vi "Find All Systems.vi"(11 "Registered Systems":T3[](array[typedef])) -> (3 "Systems":T1[](array[typedef]))   [LabVIEW 2019]
uses:
  Type Defs and Controls/Registered System.ctl
  Type Defs and Controls/System Type.ctl
  Type Defs and Controls/System Cluster.ctl
  <vilib>/nisyscfg/Find Hardware.vi
  <vilib>/nisyscfg/Close (System).vi
  <resource>/objmgr/daqmx.rc
  <vilib>/nisyscfg/nisyscfg.lvlib
  <resource>/objmgr/nicontrollersysapi.rc
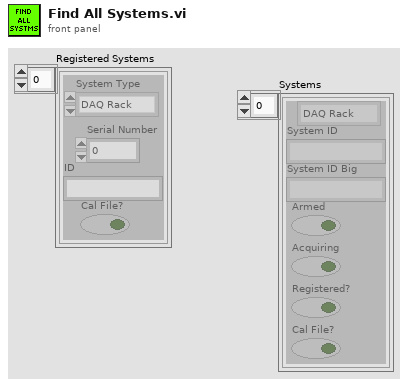
[diagram p1: front panel]
types:
  T1 = typedef "System Cluster.ctl" = cluster{"System Type":T2, "System ID":string, "System ID Big":string, "Armed":bool, "Acquiring":bool, "Registered?":bool, "Cal File?":bool}
  T2 = typedef "System Type.ctl" = enum16{"DAQ Rack", "DAQ Cart", "nx-5000", "unknown", "open"}
  T3 = typedef "Registered System.ctl" = cluster{"System Type":T2, "Serial Number":u32, "ID":string, "Cal File?":bool}
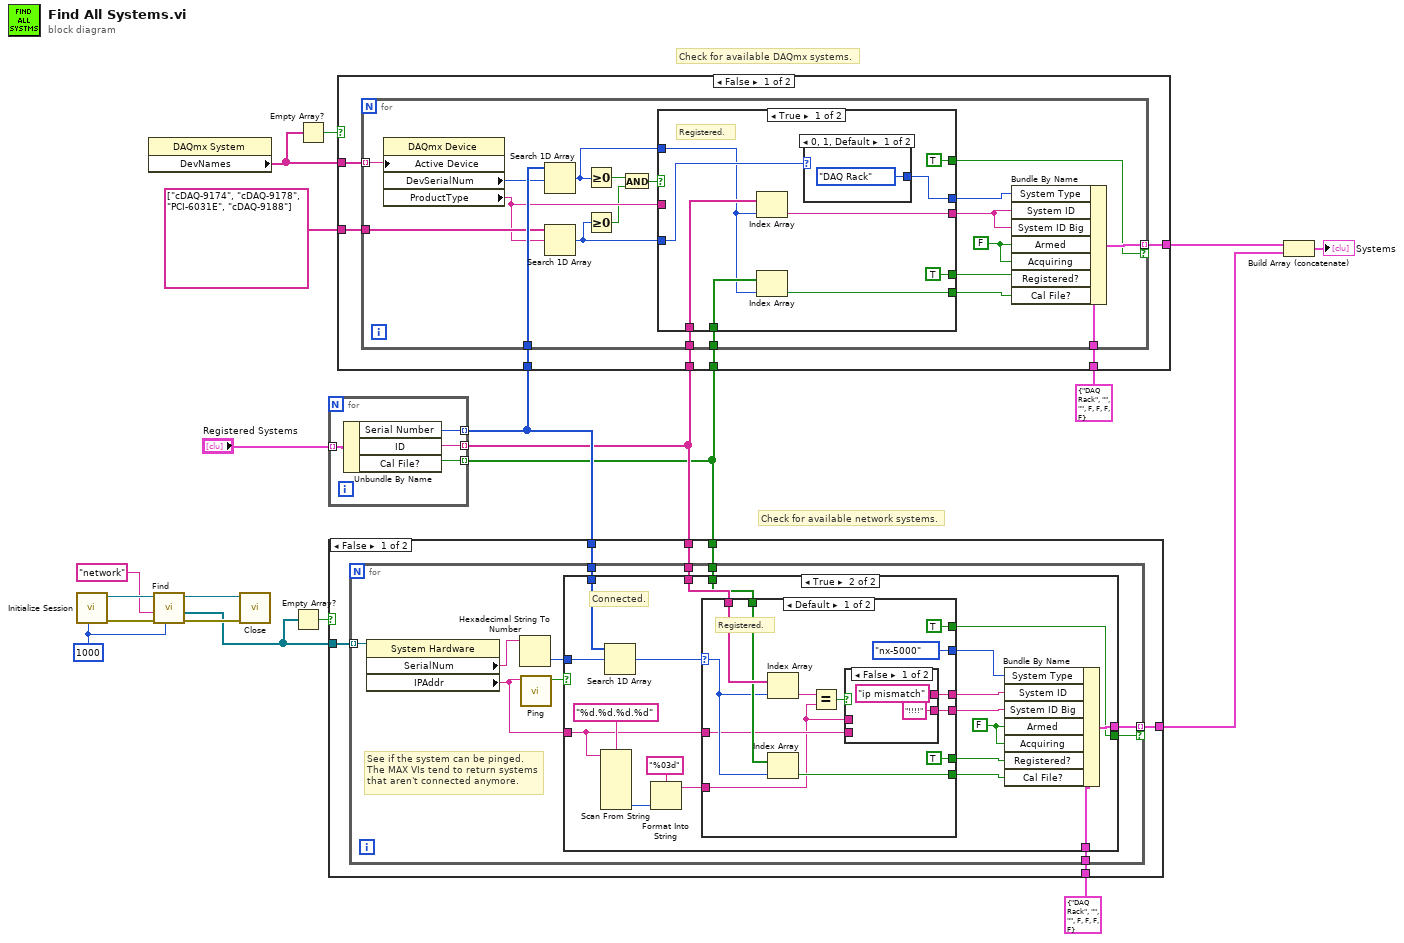
[diagram p0: block diagram]
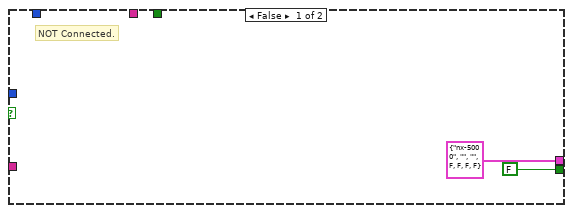
[diagram p2: hidden frame]
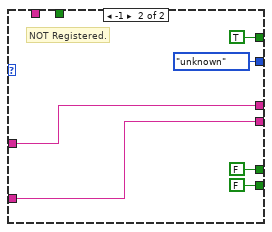
[diagram p4: hidden frame]
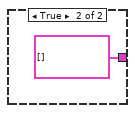
[diagram p5: hidden frame]
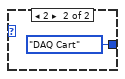
[diagram p6: hidden frame]
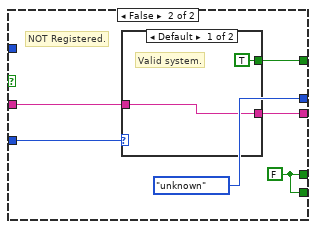
[diagram p7: hidden frame]
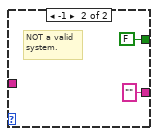
[diagram p8: hidden frame]
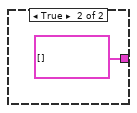
[diagram p9: hidden frame]
diagram:
  w15 = u32 1000 ("connect timeout in ms (4s)")
  # "Check for available network systems."
  # "Check for available DAQmx systems."
  n1 = call <vilib>:"Initialize Session.vi"("Connect Timeout (4000 ms)"=w15) -> ("error out"=w14:errorcluster, "Session out"=w11:refnum<k21>)  [unwired: 9 in]
  n2 = property class="DAQmx System"() -> ("DevNames"=w20:tag[])  [unwired: 2 in, 2 out]
  n3 = call-poly <vilib>:"Find.vi"("Remote Timeout (300,000 ms)"=w15, "error in (no error)"=w14, "Experts"="network" ("experts"), "Session in"=w11) -> ("error out"=w13:errorcluster, "Resources out"=w10:refnum<k20>[], "Session out"=w12:refnum<k21>)  [unwired: 4 in, 1 out]
  n4 = call-poly <vilib>:"Close.vi"("error in (no error)"=w13, "Session in"=w12) -> ()  [unwired: 9 in, 1 out]
  n5 = Empty Array?(array=w10) -> (empty?=w9:bool)
  n6 = Empty Array?(array=w20) -> (empty?=w19:bool)
  n7 = for {
    tunnel: "Registered Systems" -> [w24] mode=indexing
    tunnel: [w23] -> w8 mode=indexing
    tunnel: [w22] -> w6 mode=indexing
    tunnel: [w21] -> w5 mode=indexing
    n8 = Unbundle By Name(w24) -> ("Serial Number"=w23:u32, "ID"=w22:string, "Cal File?"=w21:bool)
  }
  n9 = case shown="False" w9 {
    tunnel: w10 -> [w30 _]
    tunnel: w8 -> [w29 _]
    tunnel: T1 {"System Type"=enum."DAQ Rack", "System ID"="", "System ID Big"="", "Armed"=FALSE, "Acquiring"=FALSE, "Registered?"=FALSE, "Cal File?"=FALSE} ("Cluster") -> [w28 _]
    tunnel: w6 -> [w27 _]
    tunnel: w5 -> [w26 _]
    tunnel: [w25 T1[] []] -> w3
    frame False {
      n10 = for {
        tunnel: w30 -> [w41] mode=indexing
        tunnel: w29 -> [w37]
        tunnel: w28 -> [w36]
        tunnel: w27 -> [w35]
        tunnel: w26 -> [w34]
        tunnel: [w33] -> w25 mode=indexing if=w32
        # "See if the system can be pinged.\nThe MAX VIs tend to return systems\nthat aren't connected anymore."
        n11 = property class="System Hardware"(reference=w41) -> ("SerialNum"=w39:string, "IPAddr"=w31:string)  [unwired: 1 in, 2 out]
        n12 = Hexadecimal String To Number(string=w39) -> (number=w38:u32)  [unwired: 2 in, 1 out]
        n13 = call "Ping.vi"("IP Address"=w31) -> ("Available?"=w40:bool)  [unwired: 10 in]
        n14 = case shown="True" w40 {
          tunnel: w38 -> [_ w61]
          tunnel: w37 -> [_ w62]
          tunnel: w36 -> [_ w59]
          tunnel: w35 -> [_ w57]
          tunnel: w34 -> [_ w55]
          tunnel: [T1 {"System Type"=enum."nx-5000", "System ID"="", "System ID Big"="", "Armed"=FALSE, "Acquiring"=FALSE, "Registered?"=FALSE, "Cal File?"=FALSE} ("Cluster") w52] -> w33
          tunnel: [FALSE ("Armed") w51] -> w32
          tunnel: w31 -> [_ w48]
          frame False {
            # "NOT Connected."
          }
          frame True {
            w58 = FALSE ("Armed")
            # "Connected."
            n15 = Scan From String(format string="%d.%d.%d.%d", input string=w48) -> (output 4=w46:i32)  [unwired: 9 in, 3 out]
            n16 = Search 1D Array(1D array=w62, element=w61) -> (index of element=w60:i32)  [unwired: 1 in]
            n17 = Format Into String(format string="%03d", w46) -> (resulting string=w44:string)  [unwired: 2 in, 1 out]
            n18 = case shown="Default" w60 {
              selector: w60 -> [w73 _]
              tunnel: w57 -> [w75 _]
              tunnel: [w67 w82] -> w56
              tunnel: w55 -> [w74 _]
              tunnel: [w72 FALSE ("Cal File?")] -> w54
              tunnel: [TRUE ("Armed") FALSE ("Armed")] -> w53
              tunnel: [TRUE ("Armed") TRUE ("Armed")] -> w51
              tunnel: [w65 w80] -> w50
              tunnel: w48 -> [w66 w82]
              tunnel: [System_Type."nx-5000" ("System Type") System_Type."unknown" ("System Type")] -> w47
              tunnel: w44 -> [w63 w80]
              frame Default {
                # "Registered."
                n19 = Index Array(array=w75, index=w73) -> (element=w69:string)
                n20 = Index Array(array=w74, index=w73) -> (element=w72:bool)
                n21 = Equal?(x=w69, y=w63) -> (x = y?=w68:bool)
                n22 = case shown="False" w68 {
                  tunnel: ["ip mismatch" ("IPAddr") w79] -> w67
                  tunnel: w66 -> [_ w79]
                  tunnel: ["!!!!" w78] -> w65
                  tunnel: w63 -> [_ w78]
                  frame False {
                  }
                  frame True {
                  }
                }
              }
              frame -1 {
                # "NOT Registered."
              }
            }
            n23 = Bundle By Name(cluster=w59, "System Type"=w47, "System ID"=w56, "System ID Big"=w50, "Armed"=w58, "Acquiring"=w58, "Registered?"=w53, "Cal File?"=w54) -> (w52:T1)
          }
        }
      }
    }
    frame True {
    }
  }
  n24 = case shown="False" w19 {
    tunnel: w20 -> [w93 _]
    tunnel: string[] ["cDAQ-9174", "cDAQ-9178", "PCI-6031E", "cDAQ-9188"] -> [w92 _]
    tunnel: w8 -> [w91 _]
    tunnel: T1 {"System Type"=enum."DAQ Rack", "System ID"="", "System ID Big"="", "Armed"=FALSE, "Acquiring"=FALSE, "Registered?"=FALSE, "Cal File?"=FALSE} ("Cluster") -> [w90 _]
    tunnel: w6 -> [w89 _]
    tunnel: w5 -> [w88 _]
    tunnel: [w87 T1[] []] -> w4
    frame False {
      n25 = for {
        tunnel: w93 -> [w113] mode=indexing
        tunnel: w92 -> [w101]
        tunnel: w91 -> [w112]
        tunnel: w90 -> [w110]
        tunnel: w89 -> [w109]
        tunnel: w88 -> [w105]
        tunnel: [w103] -> w87 mode=indexing if=w102
        w107 = FALSE ("Armed")
        n26 = property class="DAQmx Device"("Active Device"=w113) -> ("DevSerialNum"=w111:u32, "ProductType"=w99:string)  [unwired: 2 in, 2 out]
        n27 = Search 1D Array(1D array=w112, element=w111) -> (index of element=w98:i32)  [unwired: 1 in]
        n28 = Search 1D Array(1D array=w101, element=w99) -> (index of element=w97:i32)  [unwired: 1 in]
        n29 = Greater Or Equal To 0?(x=w98) -> (x >= 0?=w96:bool)
        n30 = Greater Or Equal To 0?(x=w97) -> (x >= 0?=w95:bool)
        n31 = And(x=w96, y=w95) -> (x .and. y?=w94:bool)
        n32 = case shown="True" w94 {
          tunnel: w109 -> [w122 _]
          tunnel: [w121 w128] -> w108
          tunnel: [TRUE ("Armed") w129] -> w106
          tunnel: w105 -> [w119 _]
          tunnel: [w118 w129] -> w104
          tunnel: [TRUE w130] -> w102
          tunnel: w99 -> [_ w127]
          tunnel: w97 -> [w116 w126]
          tunnel: [w115 System_Type."unknown" ("System Type")] -> w100
          tunnel: w98 -> [w114 _]
          frame True {
            # "Registered."
            n33 = Index Array(array=w122, index=w114) -> (element=w121:string)
            n34 = Index Array(array=w119, index=w114) -> (element=w118:bool)
            n35 = case shown="0, 1, Default" w116 {
              tunnel: [System_Type."DAQ Rack" ("System Type") System_Type."DAQ Cart" ("System Type")] -> w115
              frame 0, 1, Default {
              }
              frame 2 {
              }
            }
          }
          frame False {
            w129 = FALSE ("Armed")
            # "NOT Registered."
            n36 = case shown="Default" w126 {
              tunnel: [TRUE ("Armed") FALSE ("Armed")] -> w130
              tunnel: [w131 ""] -> w128
              tunnel: w127 -> [w131 _]
              frame Default {
                # "Valid system."
              }
              frame -1 {
                # "NOT a valid\nsystem."
              }
            }
          }
        }
        n37 = Bundle By Name(cluster=w110, "System Type"=w100, "System ID"=w108, "System ID Big"=w108, "Armed"=w107, "Acquiring"=w107, "Registered?"=w106, "Cal File?"=w104) -> (w103:T1)
      }
    }
    frame True {
    }
  }
  n38 = Build Array (concatenate)(w4, w3) -> (→"Systems":T1[])
